vi "setTensao.vi"(7 "Ponto":i32, 8 "error in (no error)":errorcluster, 9 "Pontos":dbl, 10 "Tensão máxima":dbl, 11 "delay(ms)":dbl) -> (0 "error out":errorcluster, 2 "output voltage":dbl)   [LabVIEW 2012]
uses:
  <instrlib>/Agilent 6XXX Series/Agilent 6XXX Series.lvlib
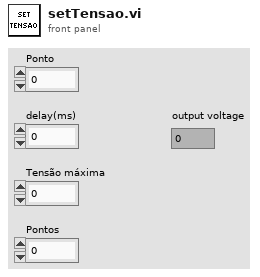
[diagram p1: front panel]
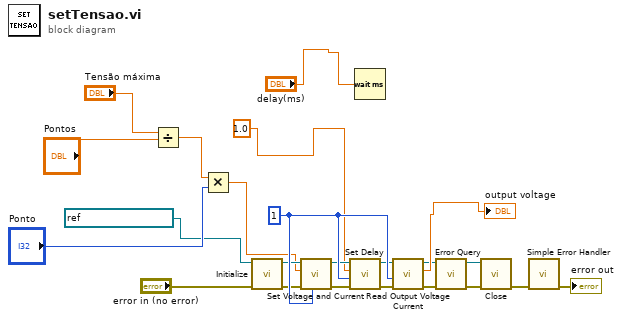
[diagram p0: block diagram]
diagram:
  w19 = u8 1 ("channel (1)")
  n1 = Divide(x="Tensão máxima", y="Pontos") -> (x/y=w18:dbl)
  n2 = Multiply(x=w18, y="Ponto") -> (x*y=w6:dbl)
  n3 = call <instrlib>:"Initialize.vi"("error in (no error)"="error in (no error)", "VISA resource name"=refnum<visa-resource-name> "GPIB0::5::INSTR") -> ("error out"=w12:errorcluster, "VISA resource name out"=w13:refnum<visa-resource-name>)  [unwired: 8 in]
  n4 = call <instrlib>:"Set Voltage and Current.vi"("channel (1)"=w19, "error in (no error)"=w12, "voltage (0 V)"=w6, "VISA resource name"=w13) -> ("error out"=w8:errorcluster, "VISA resource name out"=w7:refnum<visa-resource-name>)  [unwired: 6 in]
  n5 = call <instrlib>:"Set Delay.vi"("error in (no error)"=w8, "channel (1)"=w19, "delay (0 s)"=1.0, "VISA resource name"=w7) -> ("error out"=w4:errorcluster, "VISA resource name out"=w5:refnum<visa-resource-name>)  [unwired: 6 in]
  n6 = Wait (ms)(milliseconds to wait="delay(ms)") -> ()  [unwired: 1 out]
  n7 = call <instrlib>:"Read Output Voltage Current.vi"("error in (no error)"=w4, "channel (1)"=w19, "VISA resource name"=w5) -> ("error out"=w10:errorcluster, "output voltage"=→"output voltage":dbl, "VISA resource name out"=w9:refnum<visa-resource-name>)  [unwired: 5 in, 1 out]
  n8 = call <instrlib>:"Error Query.vi"("error in (no error)"=w10, "VISA resource name"=w9) -> ("error out"=w15:errorcluster, "VISA resource name out"=w14:refnum<visa-resource-name>)  [unwired: 6 in, 2 out]
  n9 = call <instrlib>:"Close.vi"("error in (no error)"=w15, "VISA resource name"=w14) -> ("error out"=w16:errorcluster)  [unwired: 9 in]
  n10 = call <vilib>:"Simple Error Handler.vi"("error in (no error)"=w16) -> ("error out"=→"error out":errorcluster)  [unwired: 4 in, 4 out]
